vi "UMLEditor_GetAllClassNodeNames.vi"(8 "error in":errorcluster, 11 "graph":refnum<class "Graph.lvclass">) -> (0 "error out":errorcluster, 2 "ClassNodeNames(WithoutStereotype)":string[](array[string]))   [LabVIEW 2014]
uses:
  <resource>/Framework/Providers/Open_GDS/UML/Graph_class/Graph.lvclass
  <resource>/Framework/Providers/Open_GDS/UML/ClassNode_class/ClassNode.lvclass
  <resource>/Framework/Providers/Open_GDS/UML/AbstractNode_class/AbstractNode.lvclass
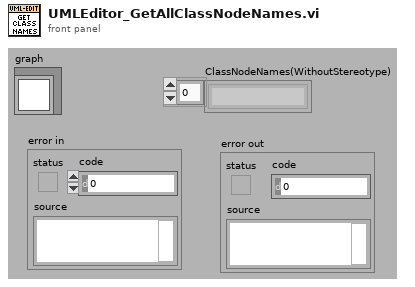
[diagram p1: front panel]
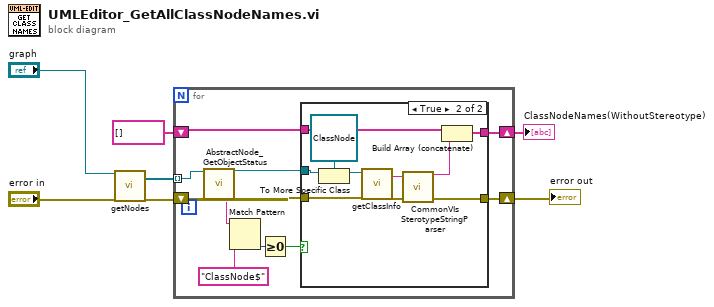
[diagram p0: block diagram]
diagram:
  n1 = call-dynamic "getNodes.vi"("reference"="graph", "error in (no error)"="error in") -> ("nodes"=w7:refnum<class "AbstractNode.lvclass">[], "error out"=w4:errorcluster)  [unwired: 15 in, 1 out]
  n2 = for {
    shift-right: [w10] -> w3
    shift-left: w4 -> [w18]
    tunnel: w7 -> [w14] mode=indexing
    shift-right: [w9] -> w1
    shift-left: string[] [] -> [w8]
    n3 = call <resource>:"AbstractNode_GetObjectStatus.vi"("reference in"=w14, "error in (no error)"=w18) -> ("Class name"=w17:string, "reference out"=w11:refnum<class "AbstractNode.lvclass">, "error out"=w12:errorcluster)  [unwired: 15 out]
    n4 = Match Pattern(string=w17, regular expression="ClassNode$") -> (offset past match=w15:i32)  [unwired: 4 out]
    n5 = Greater Or Equal To 0?(x=w15) -> (x >= 0?=w13:bool)
    n6 = case shown="True" w13 {
      tunnel: w12 -> [w20 w29]
      tunnel: w11 -> [_ w23]
      tunnel: [w20 w28] -> w10
      tunnel: [w19 w27] -> w9
      tunnel: w8 -> [w19 w26]
      frame False {
      }
      frame True {
        n7 = To More Specific Class(target class=refnum<class "ClassNode.lvclass"> refnum ("reference"), reference=w23) -> (specific class reference=w21:refnum<class "ClassNode.lvclass">)  [unwired: 1 in, 1 out]
        n8 = call-dynamic "getClassInfo.vi"("reference"=w21, "error in (no error)"=w29) -> ("className"=w25:string, "error out"=w28:errorcluster)  [unwired: 8 in, 8 out]
        n9 = call <resource>:"CommonVIs SterotypeStringParser.vi"("SterotypeStringIn"=w25) -> ("Name"=w24:string)  [unwired: 18 out]
        n10 = Build Array (concatenate)(w26, w24) -> (w27:string[])
      }
    }
  }
  "error out" <- w3
  "ClassNodeNames(WithoutStereotype)" <- w1
